vi "Format Extended Error Info.vi"(10 "DQMH Error Hint":string, 11 "Call Chain":string[](array[string])) -> (3 "Call Chain String":string)   [LabVIEW 2016, in "hse-logger.lvlib" / "HSE_v2_Formatter.lvclass"]
uses:
  HSE_v2_Formatter.lvclass
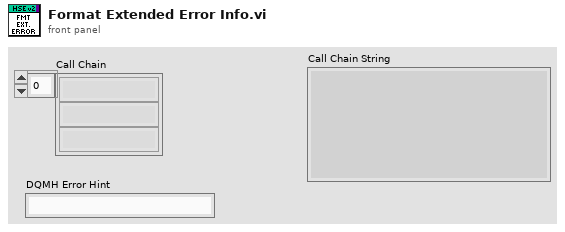
[diagram p1: front panel]
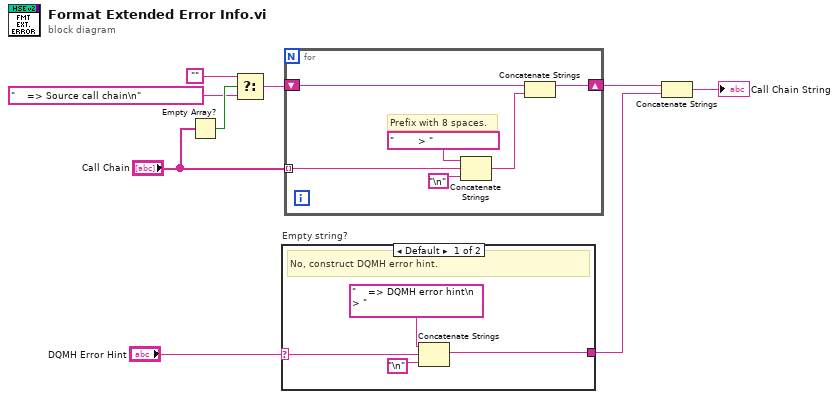
[diagram p0: block diagram]
diagram:
  n1 = Empty Array?(array="Call Chain") -> (empty?=w8:bool)
  n2 = Select(t="", s=w8, f="    => Source call chain\n") -> (s? t:f=w7:string)
  n3 = case "Empty string?" shown="Default" "DQMH Error Hint" {
    selector: "DQMH Error Hint" -> [w12 w14]
    tunnel: [w11 w14] -> w1
    frame Default {
      # "No, construct DQMH error hint."
      n4 = Concatenate Strings("    => DQMH error hint\n        > ", w12, "\n") -> (w11:string)
    }
    frame "" {
      # "Yes, do nothing."
    }
  }
  n5 = for {
    tunnel: "Call Chain" -> [w19] mode=indexing
    shift-right: [w16] -> w3
    shift-left: w7 -> [w18]
    # "Prefix with 8 spaces."
    n6 = Concatenate Strings("        > " ("string"), w19, "\n") -> (w17:string)
    n7 = Concatenate Strings(w18, w17) -> (w16:string)
  }
  n8 = Concatenate Strings(w3, w1) -> (→"Call Chain String":string)
